vi "BRig_dataRT_stats__BTPR_cur.vi"() -> (2 "output_BTPR_cur":i32)   [LabVIEW 2014]
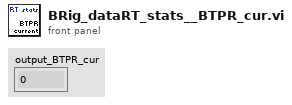
[diagram p1: front panel]
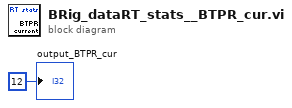
[diagram p0: block diagram]
diagram:
  "output_BTPR_cur" <- 12 ("output_iBlock")
